vi "HF modbus rtu.vi"(4 "State":i16, 5 "Time":dbl format="%.2f", 6 "Sensor Values":dbl[](array[numeric]), 7 "Set Points":dbl[](array[numeric])=[1.0]) -> (0 "required data":T1={"Set Point names"=["unitID (usually 1)", "com port number"], "required number of setpoints"=2, "required number of sensors"=0, "Sensor names"=[]}, 3 "output value":dbl)   [LabVIEW 2015]
panel:
  in  "error in (no error)":errorcluster
  # "Enter the correct information for this control code in the required data structure below. Then make the current value default by right clicking on the border of the data structure. Select \"data operations\" and then select \"make current value default\". These values will be displayed by process controller."
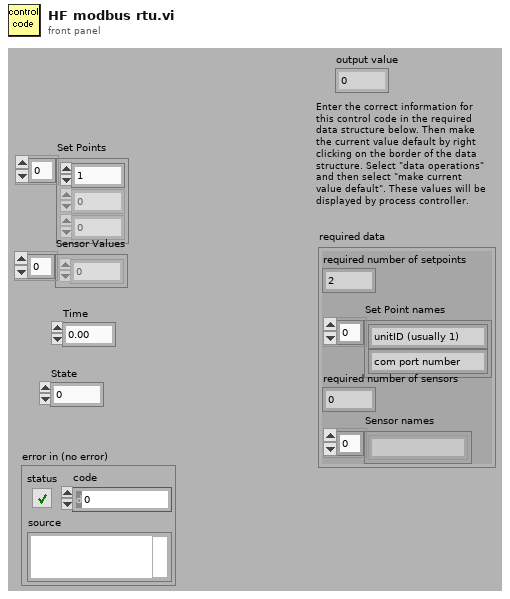
[diagram p1: front panel]
types:
  T1 = cluster{"Set Point names":string[], "required number of setpoints":u8, "required number of sensors":u8, "Sensor names":string[]}
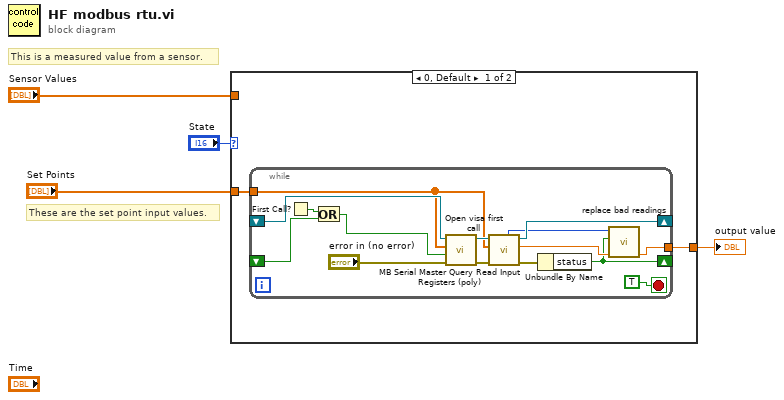
[diagram p0: block diagram]
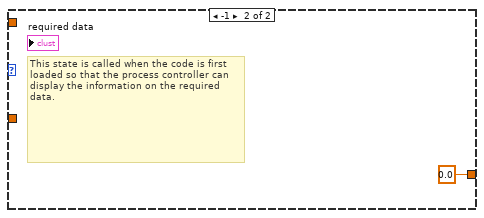
[diagram p2: hidden frame]
diagram:
  # "These are the set point input values."
  # "This is a measured value from a sensor."
  n1 = case shown="0, Default" "State" {
    tunnel: [w6 0.0 ("fraction on")] -> w3
    tunnel: "Set Points" -> [w5 _]
    tunnel: "Sensor Values" -> [_ _]
    frame 0, Default {
      n2 = while {
        tunnel: [w17] -> w6
        shift-right: [w13] -> _
        shift-left: _ -> [w18]
        tunnel: w5 -> [w7]
        shift-right: [w9] -> _
        shift-left: _ -> [w15]
        stop <- TRUE stop-if-true
        n3 = First Call?() -> (First Call?: T/F=w20:bool)
        n4 = Or(x=w20, y=w15) -> (x .or. y?=w16:bool)
        n5 = call "Open visa first call.vi"("error in (no error)"="error in (no error)", "First Call?: T/F"=w16, "Set Points"=w7, "VISA Refnum in"=w18) -> ("error out"=w11:errorcluster, "VISA Refnum out"=w14:refnum<visa-resource-name>)  [unwired: 6 in]
        n6 = call "MB Serial Master Query Read Input Registers (poly).vi"("error in"=w11, "Set Points"=w7, "VISA resource name"=w14) -> ("error out"=w12:errorcluster, "Meter reading"=w10:sgl, "VISA resource name out"=w13:refnum<visa-resource-name>, "Unit id"=w8:i32)  [unwired: 5 in]
        n7 = Unbundle By Name(w12) -> ("status"=w9:bool)
        n8 = call "replace bad readings.vi"("Meter reading in"=w10, "bad data read"=w9, "Unit ID"=w8) -> ("Meter reading out"=w17:dbl)  [unwired: 8 in]
      }
    }
    frame -1 {
      # "This state is called when the code is first loaded so that the process controller can display the information on the required data."
    }
  }
  "output value" <- w3
